vi "h5_1D_SGL.vi"(6 "Attributes":variant, 7 "TYPE":string, 8 "error in (no error)":errorcluster, 9 "1D SGL":sgl[](array[numeric]), 10 "SQUID":string, 11 "H5":path[](array[path])) -> (0 "error out":errorcluster, 2 "Exists":bool)   [LabVIEW 2013]
uses:
  <vilib>/addons/h5labview2/file/H5Fmode.ctl
  <vilib>/addons/h5labview2/base/lib_path.vi
  <vilib>/addons/h5labview2/base/H5Equery.vi
  <vilib>/addons/h5labview2/dataset/H5Dwrite.llb/H5Dwrite.xnode
  <vilib>/addons/h5labview2/base/hid_t.ctl
  <vilib>/addons/h5labview2/file/H5F.lvlib
  <vilib>/addons/h5labview2/dataset/H5D.lvlib
  <vilib>/addons/h5labview2/group/H5G.lvlib
  <vilib>/addons/h5labview2/space/H5S.lvlib
  <vilib>/addons/h5labview2/attrib/H5A.lvlib
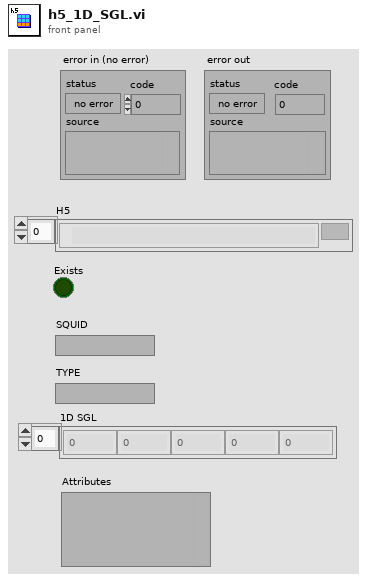
[diagram p1: front panel]
types:
  T1 = typedef "Semaphore RefNum" = refnum<k1>
  T2 = typedef "H5F.lvlib/H5Fmode.ctl" = enum16{"read-only", "read-write", "overwrite", "create new", "open or create"}
  T3 = typedef "hid_t.ctl" = i32
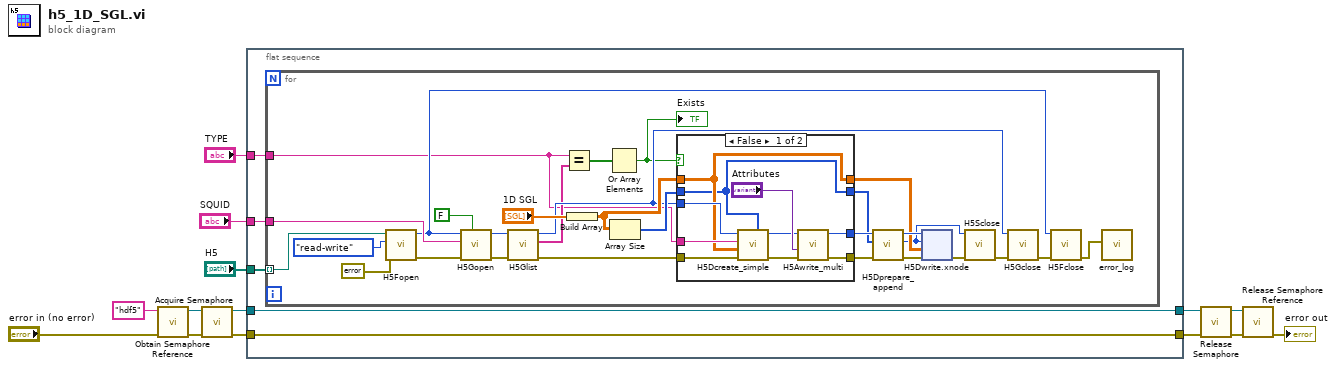
[diagram p0: block diagram]
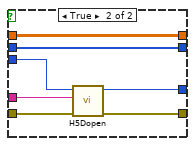
[diagram p2: hidden frame]
diagram:
  n1 = call <vilib>:"Obtain Semaphore Reference.vi"("error in (no error)"="error in (no error)", "name (unnamed)"="hdf5") -> ("error out"=w13:errorcluster, "semaphore"=w14:T1)  [unwired: 3 in, 1 out]
  n2 = call <vilib>:"Acquire Semaphore.vi"("error in (no error)"=w13, "semaphore"=w14) -> ("error out"=w7:errorcluster, "semaphore out"=w6:T1)  [unwired: 3 in, 1 out]
  n3 = flat-sequence {
    tunnel: [w19] -> w8
    tunnel: w7 -> [w19]
    tunnel: w6 -> [w18]
    tunnel: [w18] -> w5
    tunnel: "H5" -> [w17]
    tunnel: "SQUID" -> [w16]
    tunnel: "TYPE" -> [w15]
    frame #0 {
      n4 = for {
        tunnel: w17 -> [w32] mode=indexing
        tunnel: w16 -> [w33]
        tunnel: w15 -> [w24]
        n5 = call <vilib>:"H5Fopen.vi"("error in (no error)"=errorcluster {"status"=FALSE, "code"=0, "source"=""}, "mode (read-only)"=H5Fmode."read-write", "path"=w32) -> ("error out"=w31:errorcluster, "ref out"=w30:T3)  [unwired: 7 in]
        n6 = call <vilib>:"H5Gopen.vi"("create? (F)"=FALSE, "error in (no error)"=w31, "name"=w33, "ref in"=w30) -> ("error out"=w28:errorcluster, "group out"=w29:T3)  [unwired: 6 in]
        n7 = call <vilib>:"H5Glist.vi"("error in (no error)"=w28, "ref in"=w29) -> ("error out"=w27:errorcluster, "names"=w25:string[], "ref out"=w26:T3)  [unwired: 6 in, 1 out]
        n8 = Equal?(x=w24, y=w25) -> (x = y?=w23:bool[])
        n9 = Build Array("1D SGL") -> (w41:sgl[][])
        n10 = Or Array Elements(Boolean array=w23) -> (logical OR=w22:bool)
        "Exists" <- w22
        n11 = Array Size(array=w41) -> (size(s)=w42:i32[])
        n12 = case shown="False" w22 {
          tunnel: w27 -> [w76 w81]
          tunnel: w41 -> [w73 w83]
          tunnel: w26 -> [w75 w78]
          tunnel: w24 -> [w74 w79]
          tunnel: [w69 w80] -> w47
          tunnel: [w70 w77] -> w46
          tunnel: w42 -> [w72 w82]
          tunnel: [w73 w83] -> w38
          tunnel: [w72 w82] -> w40
          frame False {
            n13 = call <vilib>:"H5Dcreate_simple.vi"("chunk size"=w72, "error in (no error)"=w76, "type in"=w73, "name"=w74, "ref in"=w75) -> ("error out"=w68:errorcluster, "dset out"=w67:T3)  [unwired: 5 in]
            n14 = call <vilib>:"H5Awrite_multi.vi"("error in (no error)"=w68, "variant in"="Attributes", "ref in"=w67) -> ("error out"=w69:errorcluster, "ref out"=w70:T3)  [unwired: 7 in]
          }
          frame True {
            n15 = call <vilib>:"H5Dopen.vi"("error in (no error)"=w81, "name"=w79, "loc in"=w78) -> ("error out"=w80:errorcluster, "dset out"=w77:T3)  [unwired: 7 in]
          }
        }
        n16 = call <vilib>:"H5Dprepare_append.vi"("error in (no error)"=w47, "append dims"=w40, "dset in"=w46) -> ("error out"=w45:errorcluster, "space out"=w37:T3, "dset out"=w39:T3)  [unwired: 6 in]
        n17 = xnode "H5Dwrite.xnode"("error in (no error)"=w45, "data"=w38, "file space"=w37, "ref in"=w39) -> ("error out"=w44:errorcluster)  [unwired: 3 in, 2 out]
        n18 = call <vilib>:"H5Sclose.vi"("error in (no error)"=w44, "space in"=w37) -> ("error out"=w36:errorcluster)  [unwired: 9 in]
        n19 = call <vilib>:"H5Gclose.vi"("error in (no error)"=w36, "group in"=w26) -> ("error out"=w34:errorcluster)  [unwired: 9 in]
        n20 = call <vilib>:"H5Fclose.vi"("error in (no error)"=w34, "ref"=w30) -> ("error out"=w21:errorcluster)  [unwired: 9 in]
        n21 = call "error_log.vi"("error"=w21) -> ()  [unwired: 10 in]
      }
    }
  }
  n22 = call <vilib>:"Release Semaphore.vi"("error in (no error)"=w8, "semaphore"=w5) -> ("error out"=w9:errorcluster, "semaphore out"=w10:T1)  [unwired: 4 in]
  n23 = call <vilib>:"Release Semaphore Reference.vi"("error in (no error)"=w9, "semaphore"=w10) -> ("error out"=→"error out":errorcluster)  [unwired: 8 in, 1 out]
